vi "Leap Hand Position and Velocity.vi"() -> ()   [LabVIEW 2011, in "LVH-Leap.lvlib"]
doc: "This example demonstrates how to read the hand position and velocity using the Leap Motion Controller."
uses:
  vi.lib/LabVIEW Hacker/Leap/LVH-Leap.lvlib
  vi.lib/LabVIEW Hacker/Leap/Public/Instance VIs/Read 1 Hand Position Velocity.vi
panel:
  out "X Velocity (m/s)":sgl(slide) scale=-2.0..2.0
  out "Z Velocity (m/s)":sgl(slide) scale=2.0..-2.0
  out "Hand XZ Position":cluster{"X":sgl, "Y":sgl, "Z":sgl}
  out "Hand XZ Position":cluster{"X":sgl, "Z":sgl}[](graph)
  in  "Stop Button":bool
  # "Leap Hand Position and Velocity Example\n\nThis example demonstrates how to read the position and velocity of a hand object using the Leap Motion Controller.\n\nInstructions\n1. Connect the Leap Motion Controller to the host computer.\n2. Click the Run Arrow.\n3. Position your hand above the Leap Motion controller.  \n4. Notice your hand position and velocity indicated on the graph and sliders below."
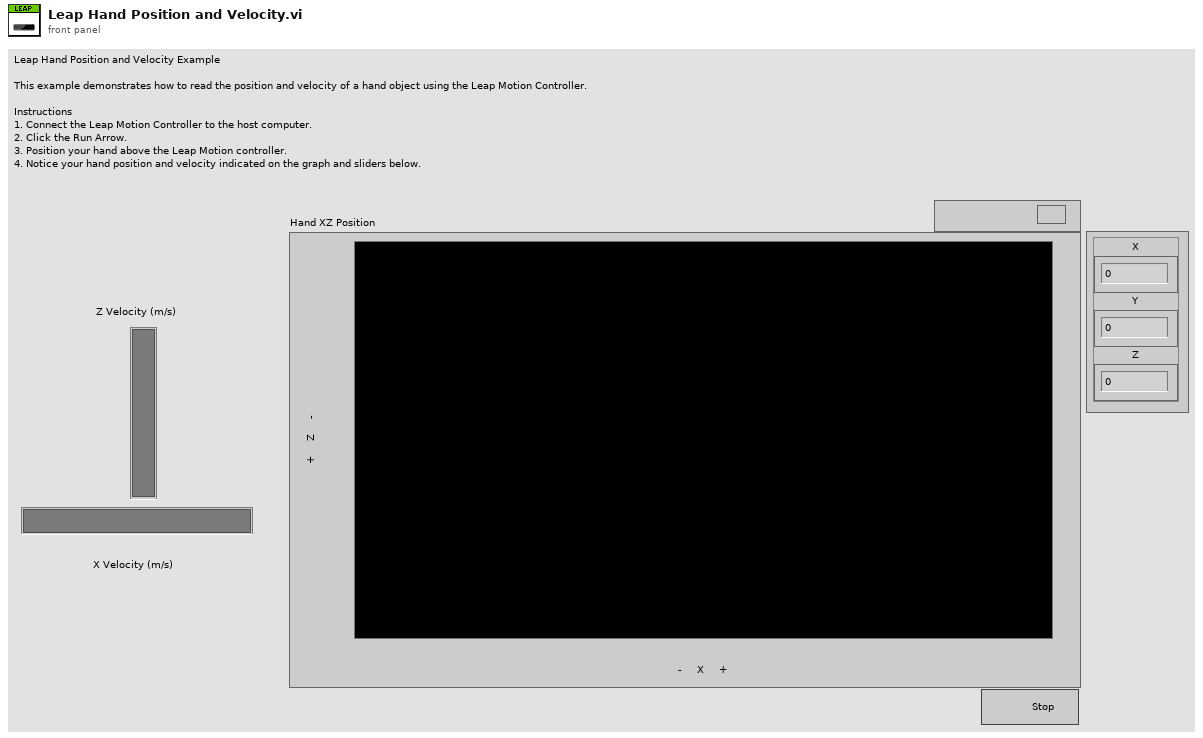
[diagram p1: front panel]
types:
  T1 = typedef "LVH-Leap.lvlib/Leap Handle.ctl" = cluster{"LeapCSharp":refnum<k24>}
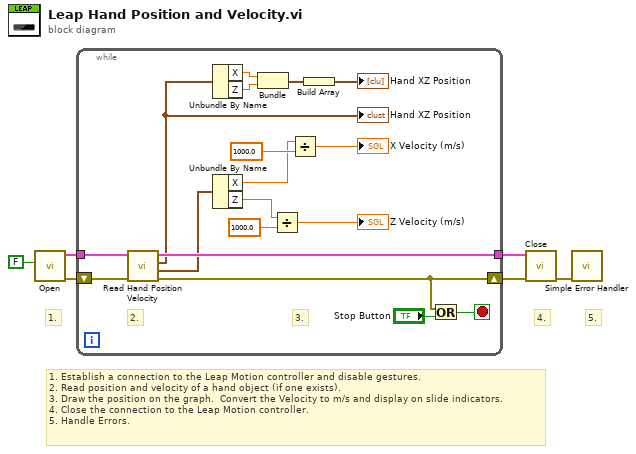
[diagram p0: block diagram]
diagram:
  # "1. Establish a connection to the Leap Motion controller and disable gestures.\n2. Read position and velocity of a hand object (if one exists).\n3. Draw the position on the graph.  Convert the Velocity to m/s and display on slide indicators.\n4. Close the connection to the Leap Motion controller.\n5. Handle Errors."
  # "5."
  # "4."
  # "1."
  n1 = call "Open.vi"("Enable Gestures? (T)"=FALSE) -> ("Error Out"=w4:errorcluster, "Leap Handle"=w6:T1)  [unwired: 9 in]
  n2 = while {
    tunnel: w6 -> [w22]
    shift-right: [w19] -> w5
    shift-left: w4 -> [w20]
    tunnel: [w21] -> w2
    stop <- w24 stop-if-true
    # "3."
    # "2."
    n3 = call-poly "Read Hand Position Velocity.vi"("Error In"=w20, "Leap Handle"=w22) -> ("Error Out"=w19:errorcluster, "Hand Velocity"=w13:cluster{"X":sgl, "Y":sgl, "Z":sgl}, "Hand Position"=w18:cluster{"X":sgl, "Y":sgl, "Z":sgl}, "Leap Handle"=w21:T1)  [unwired: 6 in]
    "Hand XZ Position" <- w18
    n4 = Unbundle By Name(w18) -> ("X"=w17:sgl, "Z"=w16:sgl)
    n5 = Unbundle By Name(w13) -> ("X"=w8:sgl, "Z"=w12:sgl)
    n6 = Bundle("X"=w17, "Z"=w16) -> (w15:cluster{"X":sgl, "Z":sgl})  [unwired: 1 in]
    n7 = Divide(x=w12, y=sgl 1000.0) -> (x/y=→"Z Velocity (m/s)":sgl)
    n8 = Divide(x=w8, y=sgl 1000.0) -> (x/y=→"X Velocity (m/s)":sgl)
    n9 = Build Array(w15) -> (→"Hand XZ Position":cluster{"X":sgl, "Z":sgl}[])
    n10 = Or(x=w19, y="Stop Button") -> (x .or. y?=w24:bool)
  }
  n11 = call "Close.vi"("Error In"=w5, "Leap Handle"=w2) -> ("Error Out"=w1:errorcluster)  [unwired: 9 in]
  n12 = call <vilib>:"Simple Error Handler.vi"("error in (no error)"=w1) -> ()  [unwired: 4 in, 5 out]
